vi "read.vi"(8 "error in (no error)":errorcluster, 10 "ILC":refnum<class "ILC.lvclass">, 11 "ReadILCLIMSW1Strategy in":refnum<class "ReadILCDCAPressure3Strategy.lvclass">) -> (0 "error out":errorcluster, 2 "Value":dbl, 3 "ReadILCLIMSW1Strategy out":refnum<class "ReadILCDCAPressure3Strategy.lvclass">)   [LabVIEW 2016, in "ReadILCDCAPressure3Strategy.lvclass"]
uses:
  ReadILCDCAPressure3Strategy.lvclass
  Common_ILC/ILC/ILC.lvclass
  Common_ILC/ILC/ILC.lvclass/ILC.ctl
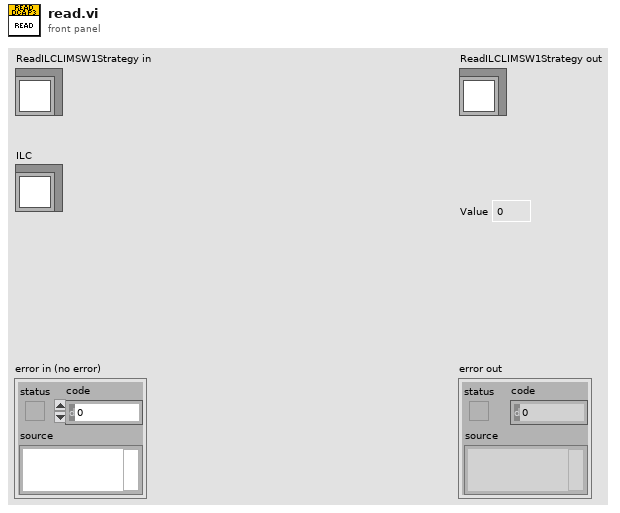
[diagram p1: front panel]
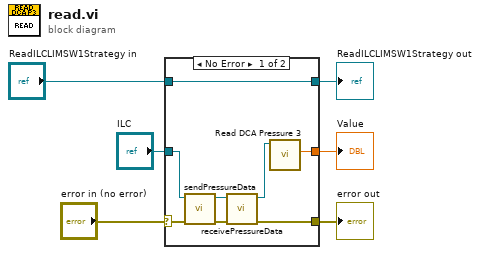
[diagram p0: block diagram]
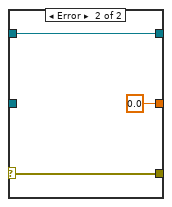
[diagram p2: hidden frame]
diagram:
  n1 = case shown="No Error" "error in (no error)" {
    selector: "error in (no error)" -> [w8 w17]
    tunnel: [w9 w17] -> w5
    tunnel: [w14 w16] -> w3
    tunnel: "ReadILCLIMSW1Strategy in" -> [w14 w16]
    tunnel: [w13 0.0 ("Value")] -> w2
    tunnel: "ILC" -> [w12 _]
    frame No Error {
      n2 = call "sendPressureData.vi"("error in (no error)"=w8, "ILC in"=w12) -> ("error out"=w7:errorcluster, "ILC out"=w11:refnum<class "ILC.lvclass">)  [unwired: 8 in]
      n3 = call "receivePressureData.vi"("error in (no error)"=w7, "ILC in"=w11) -> ("error out"=w9:errorcluster, "ILC out"=w10:refnum<class "ILC.lvclass">)  [unwired: 8 in]
      n4 = call "Read DCA Pressure 3.vi"("ILC in"=w10) -> ("DCA Pressure 3"=w13:dbl)  [unwired: 9 in, 1 out]
    }
    frame Error {
    }
  }
  "error out" <- w5
  "ReadILCLIMSW1Strategy out" <- w3
  "Value" <- w2
